vi "Actor Core.vi"(8 "error in":errorcluster, 11 "Nested in":refnum<class "Messaging Manager Actor.lvclass">) -> (0 "error out":errorcluster, 3 "Actor out":refnum<class "Actor.lvclass">)   [LabVIEW 2024, in "PCAN.lvlib" / "Messaging Manager Actor.lvlib" / "Messaging Manager Actor.lvclass"]
doc: "(<B>Filename</B>: Actor Framework.lvlib:Actor.lvclass:Actor Core.vi)\n\nReceives messages to the actor, reacts to them, and initiates any error handling that may shut the actor down.\n\nDescendant classes may override this VI to append parallel tasks for the actor to complete while it handles messages. Overrides use the Call Parent Method node."
uses:
  Messaging Manager Actor.lvclass
  Messaging Manager Actor.lvclass/Messaging Manager Actor.ctl
  <vilib>/ActorFramework/Actor/Actor.lvclass
  Messaging Buffer/Message Buffer.lvclass
  Messaging Manager Actor Messages/Read to Buffer Msg/Read to Buffer Msg.lvclass
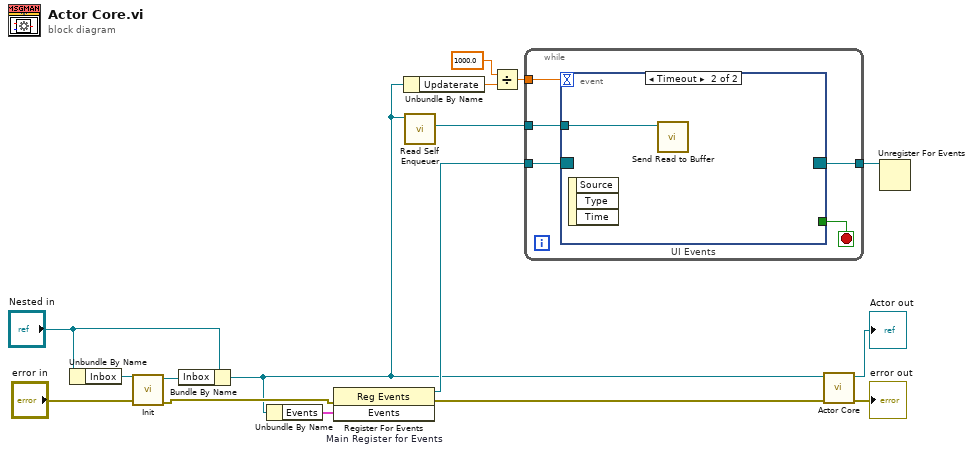
[diagram p0: block diagram]
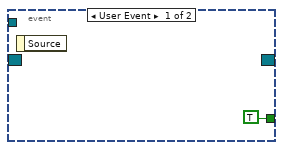
[diagram p2: hidden frame]
diagram:
  n1 = Unbundle By Name("Nested in") -> ("Inbox"=w5:refnum<class "Message Buffer.lvclass">)
  n2 = call "Init.vi"("error in"="error in", "Messaging Buffer in"=w5) -> ("error out"=w4:errorcluster, "Messaging Buffer out"=w1:refnum<class "Message Buffer.lvclass">)  [unwired: 8 in]
  n3 = Bundle By Name(cluster="Nested in", "Inbox"=w1) -> (w2:refnum<class "Messaging Manager Actor.lvclass">)
  n4 = Unbundle By Name(w2) -> ("Events"=w13:cluster{"Stop":refnum<user-event>})
  n5 = register-events "Main Register for Events"(error in=w4, w13) -> (reference out=w14:refnum<event-registration>, error out=w10:errorcluster)  [unwired: 1 in]
  n6 = Unbundle By Name(w2) -> ("Updaterate"=w9:dbl)
  n7 = call <vilib>:"Read Self Enqueuer.vi"("Actor"=w2) -> ("Self Enqueuer"=w11:refnum<class "Message Enqueuer.lvclass">)  [unwired: 10 in]
  n8 = Divide(x=1000.0, y=w9) -> (x/y=w7:dbl)
  n9 = while {
    tunnel: w14 -> [w21]
    tunnel: [w19] -> w12
    tunnel: w11 -> [w18]
    tunnel: w7 -> [w17]
    stop <- w20 stop-if-true
    n10 = event "UI Events" shown="[1] Timeout" {
      selector: w21 -> [_ _]
      dyn-events: [_ _] -> w19
      timeout: w17 -> [_ _]
      tunnel: [TRUE _] -> w20
      tunnel: w18 -> [_ w23]
      event User Event {
        n11 = event-data() -> ()  [unwired: 1 in, 1 out]
      }
      event Timeout {
        n12 = event-data() -> ()  [unwired: 1 in, 3 out]
        n13 = call "Send Read to Buffer.vi"("Message Enqueuer"=w23) -> ()  [unwired: 9 in, 2 out]
      }
    }
  }
  n14 = call-parent "Actor Core.vi"("error in"=w10, "Actor in"=w2) -> ("error out"=→"error out":errorcluster, "Actor out"=→"Actor out":refnum<class "Actor.lvclass">)  [unwired: 8 in]
  n15 = Unregister For Events(event registration refnum=w12) -> ()  [unwired: 1 in, 1 out]
